vi "stft_demodulate_low.vi"(6 "Reset":bool, 9 "Config":T2={"IO params"={"Conversion"={"Rate"=4.0, "In channels"=2, "Out channels"=4}, "Carriers"={"Phase shift"=180.0, "Levels"=[[0.8, 0.8, 0.8], [0.03, 0.03, 0.03]], "Delay samples"=73.15}}, "High rate STFT"={"Win param"=101.5, "Window type"=61, "Win order"=2, "DFT size"=64, "Channels"=[7], "Oversample"=64}, "Low rate STFT"={"Win param"=120.0, "Window type"=61, "Win order"=8, "DFT size"=64, "Channels"=[7], "Oversample"=64}, "Filtering"={"Hum"={"Frequency"=0.0, "Tc"=0.0, "Limit"=101.5, "FFT filter"=FALSE, "Detrend mode"=enum."Robust linear", "Enable"=FALSE}, "Kalman"={"Process noise"=101.5, "Measure noise"=101.5, "Unlock m noise"=101.5, "Mode"=enum."FFT"}, "Distortion"={"LF cut"=101.5, "Tc"=3.0, "Limit"=101.5, "FFT filter"=FALSE, "Detrend mode"=enum."Robust linear", "Enable"=FALSE}, "Lowpass"={"Frequency"=0.0, "Order"=0, "Enable"=FALSE}, "Impulse"={"Win order"=102, "Locked limit"=101.5, "Locked count"=102, "Threshold Tc"=101.5, "Thresh sigmas"=101.5, "Thresh min"=101.5, "After"=0, "Detrend"=FALSE, "Enable"=FALSE}}} {"Filtering"."Impulse"."Thresh min" format="%#_3p"; "Filtering"."Impulse"."Threshold Tc" format="%#_3p"; "Filtering"."Impulse"."Locked limit" format="%#_3p"; "Filtering"."Impulse"."Thresh sigmas" format="%#_3p"; "Filtering"."Lowpass"."Frequency" format="%#_4p"; "Filtering"."Distortion"."Limit" format="%#_3p"; "Filtering"."Distortion"."LF cut" format="%#_3p"; "Filtering"."Kalman"."Unlock m noise" format="%#_3p"; "Filtering"."Kalman"."Measure noise" format="%#_3p"; "Filtering"."Kalman"."Process noise" format="%#_3p"; "Filtering"."Hum"."Limit" format="%#_3p"; "Filtering"."Hum"."Frequency" format="%#_4p"; "Low rate STFT"."Oversample" min=1 step=1; "Low rate STFT"."Channels" min=0 step=1; "Low rate STFT"."DFT size" min=1 step=1; "Low rate STFT"."Window type" items=["Rectangle"=0, "Hanning"=1, "Hamming"=2, "Blackman-Harris"=3, "Exact Blackman"=4, "Blackman"=5, "Flat Top"=6, "4 Term B-Harris "=7, "7 Term B-Harris"=8, "Low Sidelobe"=9, "Blackman Nuttall"=11, "Triangle"=30, "Bartlett-Hanning"=31, "Bohman"=32, "Parzen"=33, "Welch"=34, "Kaiser"=60, "Dolph-Chebyshev"=61, "Gaussian"=62]; "High rate STFT"."Oversample" min=1 step=1; "High rate STFT"."Channels" min=0 step=1; "High rate STFT"."DFT size" min=1 step=1; "High rate STFT"."Window type" items=["Rectangle"=0, "Hanning"=1, "Hamming"=2, "Blackman-Harris"=3, "Exact Blackman"=4, "Blackman"=5, "Flat Top"=6, "4 Term B-Harris "=7, "7 Term B-Harris"=8, "Low Sidelobe"=9, "Blackman Nuttall"=11, "Triangle"=30, "Bartlett-Hanning"=31, "Bohman"=32, "Parzen"=33, "Welch"=34, "Kaiser"=60, "Dolph-Chebyshev"=61, "Gaussian"=62]; "IO params"."Carriers"."Levels" min=0.0 step=0.1; "IO params"."Conversion"."Rate" format="%#_8g"}, 10 "Modulation info":T1={"Fs full"=0.0, "Fs high"=0.0, "Fs low"=0.0, "Read size"=0, "FFT size low"=5000, "df low"=5000.0, "High carriers"=[], "Low carriers"=[], "Hi channels at low"=[7]} {"Hi channels at low" min=0 step=1; "Low carriers" format="%#_6p"; "High carriers" format="%#_6p"}, 11 "Raw data":dbl[][](array[numeric])) -> (1 "time-freq sample info":cluster{"time steps":i32, "frequency bins":i32}, 2 "STFT":cdb[][](array[numeric]) format="%#_4p")   [LabVIEW 2014]
uses:
  ilemt_config.ctl
  IO_params.ctl
  stft_params.ctl
  <vilib>/Analysis/4window.llb/windowTd.ctl
  filter_params.ctl
  detrend_mode.ctl
  modulation_info.ctl
  <vilib>/Analysis/NI_AALPro.lvlib
panel:
  # "First row is signal, second row is current reference."
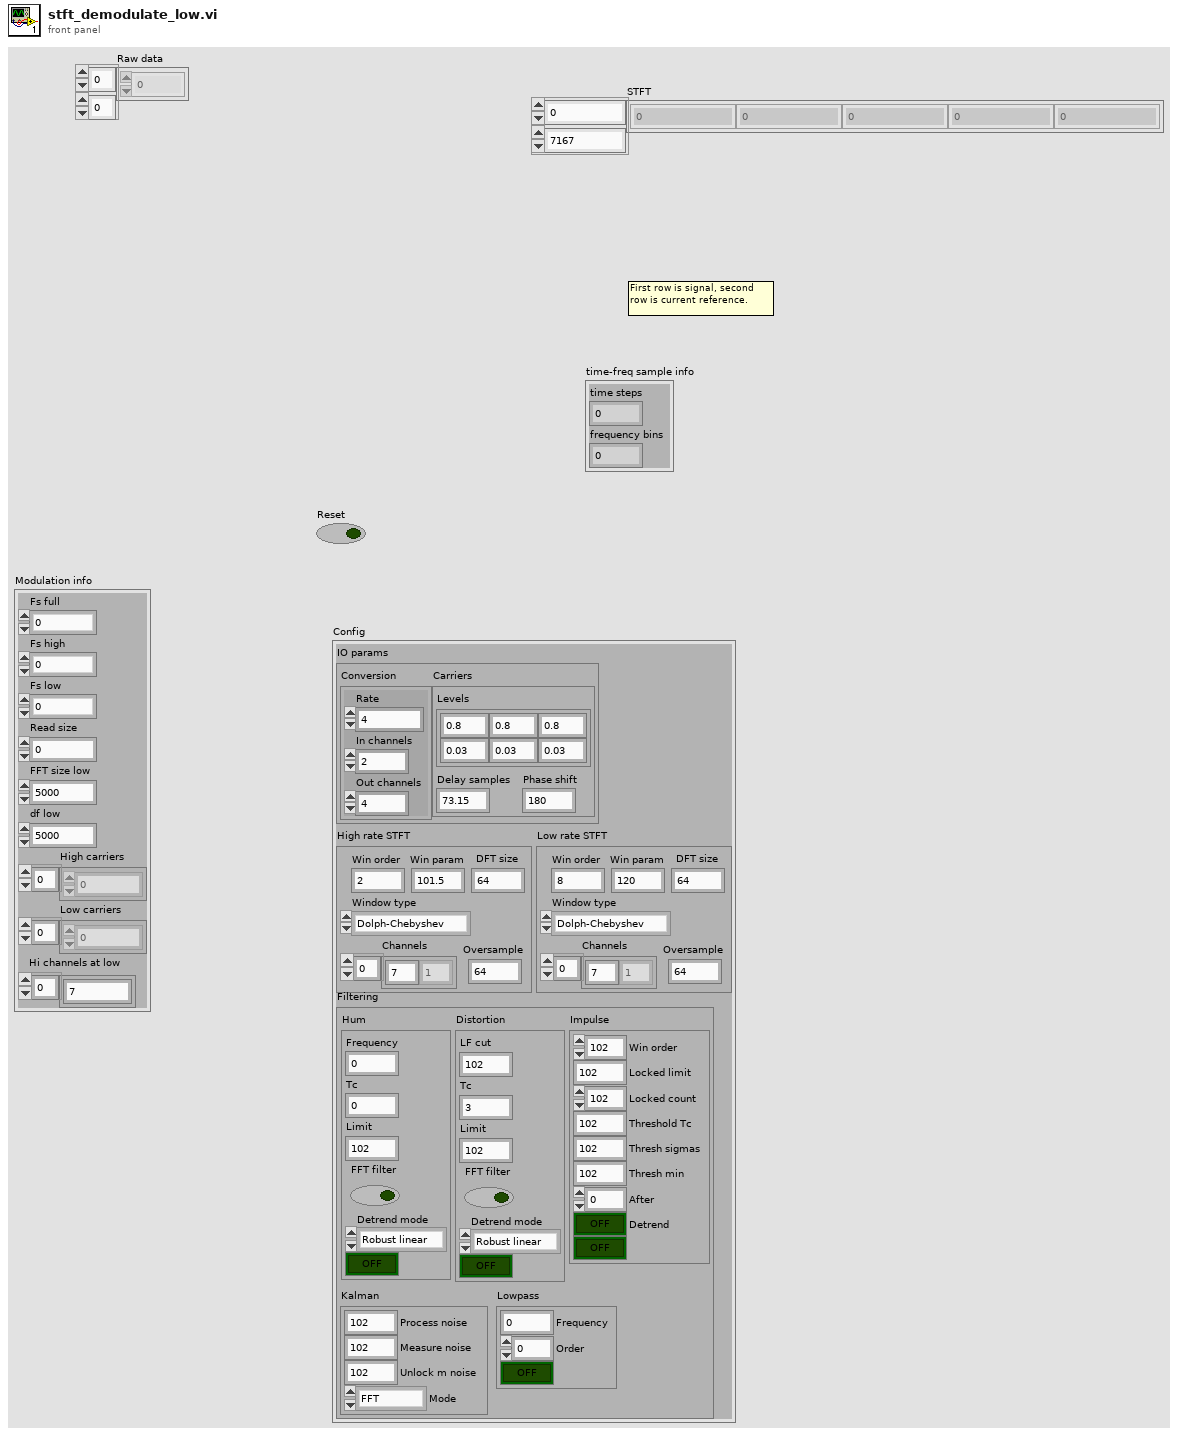
[diagram p1: front panel]
types:
  T1 = typedef "modulation_info.ctl" = cluster{"Fs full":dbl, "Fs high":dbl, "Fs low":dbl, "Read size":i32, "FFT size low":i32, "df low":dbl, "High carriers":dbl[], "Low carriers":dbl[], "Hi channels at low":i32[]}
  T2 = typedef "ilemt_config.ctl" = cluster{"IO params":T3, "High rate STFT":T4, "Low rate STFT":T4, "Filtering":T6}
  T3 = typedef "IO_params.ctl" = cluster{"Conversion":cluster{"Rate":dbl, "In channels":u32, "Out channels":u32}, "Carriers":cluster{"Phase shift":dbl, "Levels":dbl[][], "Delay samples":dbl}}
  T4 = typedef "stft_params.ctl" = cluster{"Win param":dbl, "Window type":T5, "Win order":i32, "DFT size":i32, "Channels":i32[], "Oversample":i32}
  T5 = typedef "NI_AALPro.lvlib/windowTd.ctl" = u32
  T6 = typedef "filter_params.ctl" = cluster{"Hum":cluster{"Frequency":dbl, "Tc":dbl, "Limit":dbl, "FFT filter":bool, "Detrend mode":T7, "Enable":bool}, "Kalman":cluster{"Process noise":dbl, "Measure noise":dbl, "Unlock m noise":dbl, "Mode":enum16{"FFT", "KF demod"}}, "Distortion":cluster{"LF cut":dbl, "Tc":dbl, "Limit":dbl, "FFT filter":bool, "Detrend mode":T7, "Enable":bool}, "Lowpass":cluster{"Frequency":dbl, "Order":i32, "Enable":bool}, "Impulse":cluster{"Win order":i32, "Locked limit":dbl, "Locked count":i32, "Threshold Tc":dbl, "Thresh sigmas":dbl, "Thresh min":dbl, "After":i32, "Detrend":bool, "Enable":bool}}
  T7 = typedef "detrend_mode.ctl" = enum16{"Zero mean", "Linear", "Robust linear"}
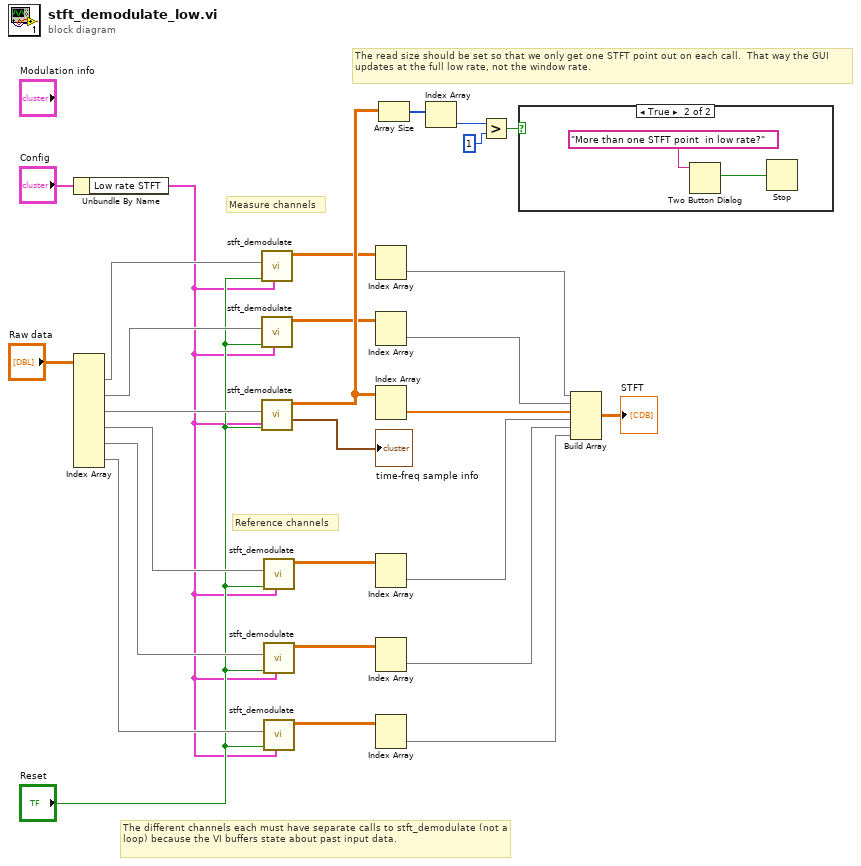
[diagram p0: block diagram]
diagram:
  # "The different channels each must have separate calls to stft_demodulate (not a loop) because the VI buffers state about past input data."
  # "Reference channels"
  # "Measure channels"
  # "The read size should be set so that we only get one STFT point out on each call.  That way the GUI updates at the full low rate, not the window rate."
  n1 = Unbundle By Name("Config") -> ("Low rate STFT"=w1:T4)
  n2 = Index Array(array="Raw data") -> (element #1=w2:dbl[], element #2=w8:dbl[], element #3=w17:dbl[], element #4=w16:dbl[], element #5=w12:dbl[], element #6=w11:dbl[])  [unwired: 12 in]
  n3 = call "stft_demodulate.vi"("STFT params"=w1, "Reset"="Reset", "X"=w2) -> ("STFT"=w6:cdb[][])  [unwired: 6 in, 2 out]
  n4 = call "stft_demodulate.vi"("STFT params"=w1, "Reset"="Reset", "X"=w8) -> ("STFT"=w5:cdb[][])  [unwired: 6 in, 2 out]
  n5 = call "stft_demodulate.vi"("STFT params"=w1, "Reset"="Reset", "X"=w17) -> ("time-freq sample info"=→"time-freq sample info":cluster{"time steps":i32, "frequency bins":i32}, "STFT"=w22:cdb[][])  [unwired: 6 in, 1 out]
  n6 = call "stft_demodulate.vi"("STFT params"=w1, "Reset"="Reset", "X"=w16) -> ("STFT"=w19:cdb[][])  [unwired: 6 in, 2 out]
  n7 = call "stft_demodulate.vi"("STFT params"=w1, "Reset"="Reset", "X"=w12) -> ("STFT"=w14:cdb[][])  [unwired: 6 in, 2 out]
  n8 = call "stft_demodulate.vi"("STFT params"=w1, "Reset"="Reset", "X"=w11) -> ("STFT"=w13:cdb[][])  [unwired: 6 in, 2 out]
  n9 = Index Array(array=w6) -> (element=w4:cdb[])  [unwired: 2 in]
  n10 = Index Array(array=w5) -> (element=w3:cdb[])  [unwired: 2 in]
  n11 = Index Array(array=w22) -> (element=w21:cdb[])  [unwired: 2 in]
  n12 = Index Array(array=w19) -> (element=w18:cdb[])  [unwired: 2 in]
  n13 = Index Array(array=w14) -> (element=w10:cdb[])  [unwired: 2 in]
  n14 = Index Array(array=w13) -> (element=w9:cdb[])  [unwired: 2 in]
  n15 = Array Size(array=w22) -> (size(s)=w26:i32[])
  n16 = Index Array(array=w26) -> (element=w25:i32)  [unwired: 1 in]
  n17 = Greater?(x=w25, y=1 ("x")) -> (0:w23:bool)
  n18 = case shown="True" w23 {
    frame False {
    }
    frame True {
      n19 = Two Button Dialog(message="More than one STFT point  in low rate?") -> (T button?=w29:bool)  [unwired: 2 in]
      n20 = Stop(stop? (T)=w29) -> ()
    }
  }
  n21 = Build Array(w4, w3, w21, w18, w10, w9) -> (→"STFT":cdb[][])
